vi "Write Number Of Dimensions.vi"(8 "error in (no error)":errorcluster, 10 "NumDims":u32, 11 "Array.lvclass in":refnum<class "Array.lvclass">) -> (0 "error out":errorcluster, 3 "Array.lvclass out":refnum<class "Array.lvclass">)   [LabVIEW 2015, in "Array.lvclass"]
uses:
  Array.lvclass
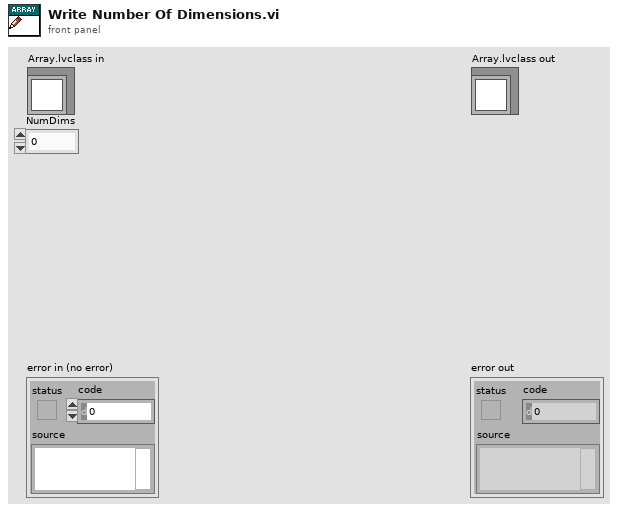
[diagram p1: front panel]
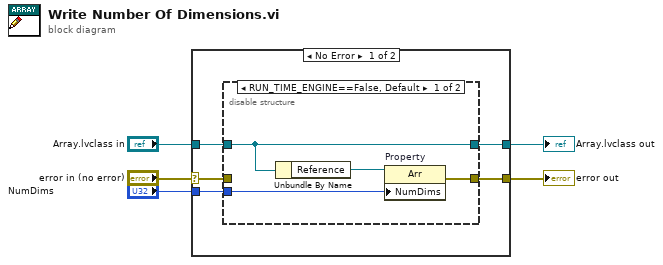
[diagram p0: block diagram]
diagram:
  n1 = case shown="No Error" "error in (no error)" {
    selector: "error in (no error)" -> [w6 w18]
    tunnel: [w10 w18] -> w4
    tunnel: [w7 w17] -> w2
    tunnel: "Array.lvclass in" -> [w8 w17]
    tunnel: "NumDims" -> [w9 _]
    frame No Error {
      n2 = disable-structure shown="RUN_TIME_ENGINE==False, Default" {
        disable-tunnel: [w14 w15] -> w10
        disable-tunnel: w9 -> [w13 _]
        disable-tunnel: w8 -> [w11 w16]
        disable-tunnel: [w11 w16] -> w7
        disable-tunnel: w6 -> [_ w15]
        frame condition #0 (active) {
          n3 = Unbundle By Name(w11) -> ("Reference"=w12:refnum<vi>)
          n4 = property on="Property" class="Arr"(reference=w12, "NumDims"=w13) -> (error out=w14:errorcluster)  [unwired: 1 in, 1 out]
        }
        frame condition #1 {
        }
      }
    }
    frame Error {
    }
  }
  "error out" <- w4
  "Array.lvclass out" <- w2
